vi "SSS_simulator.vi"() -> ()   [LabVIEW 2017]
panel:
  out "불리언":bool
  out "크기":i32
  out "배열":i32[](array[numeric])
  out "CMD_PWD_DATA":i32
  out "CMD_TVG_DATA":i32
  out "CMD_GAIN_DATA":i32
  out "CMD_RANGE_DATA":i32
  out "CMD_STOP_DATA":i32
  out "CMD_START_DATA":i32
  out "CMD_PWD":i32
  out "CMD_TVG":i32
  out "CMD_GAIN":i32
  out "CMD_RANGE":i32
  out "CMD_STOP":i32
  out "CMD_START":i32
  in  "port":u16=2500
  in  "address":string="30.0.1.18"
  in  "Server Closed":string="The server VI closed the connection."
  in  "TCP_Stop":bool
  # "TCP_Stop"
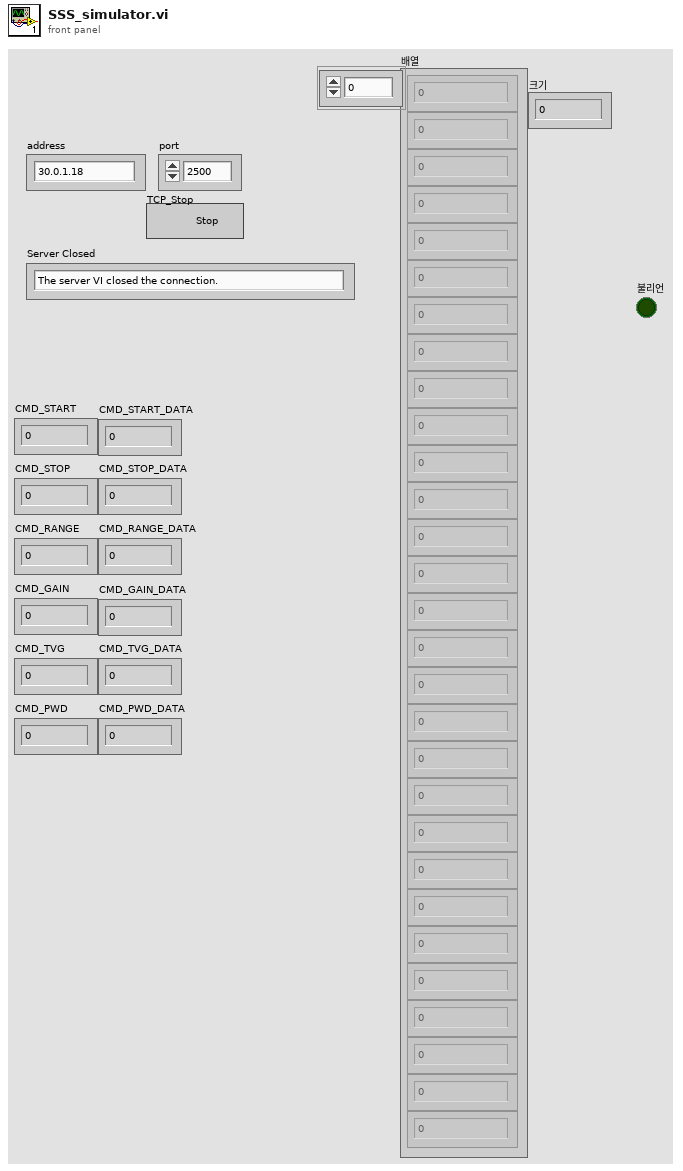
[diagram p1: front panel]
types:
  T1 = enum16{"Standard", "Buffered", "CRLF", "Immediate"}
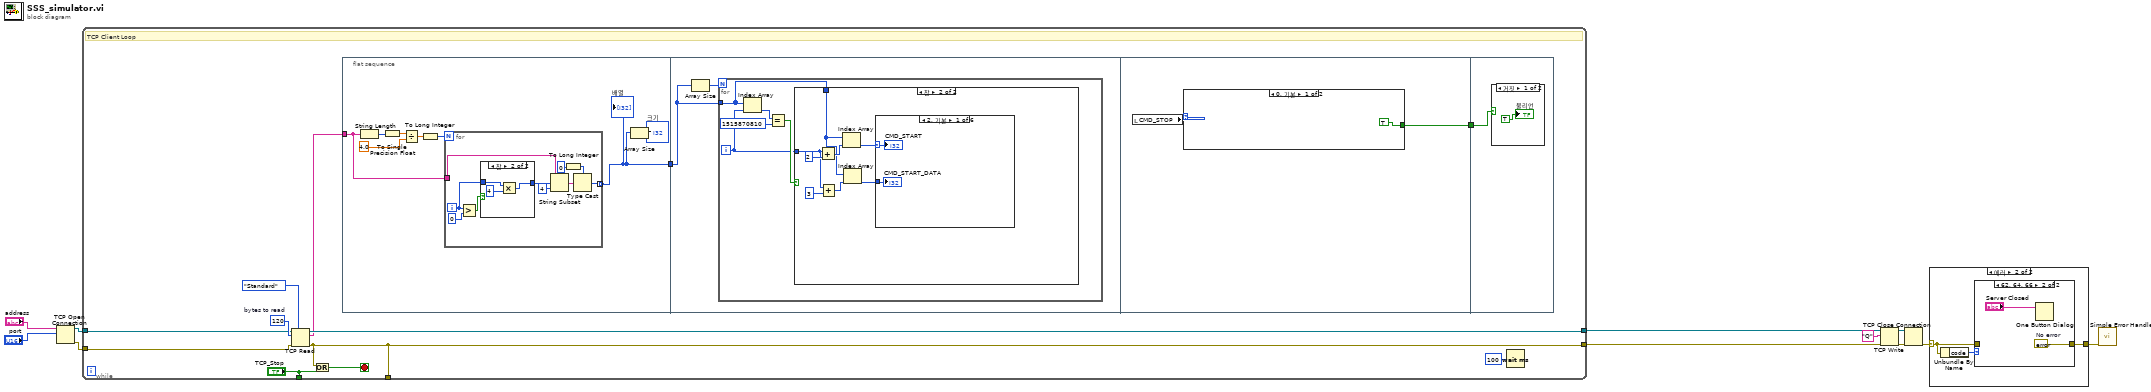
[diagram p0: block diagram]
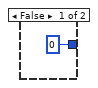
[diagram p2: hidden frame]
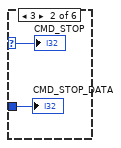
[diagram p4: hidden frame]
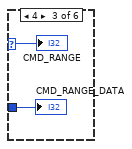
[diagram p5: hidden frame]
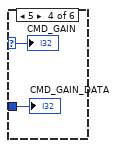
[diagram p6: hidden frame]
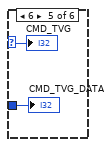
[diagram p7: hidden frame]
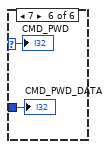
[diagram p8: hidden frame]
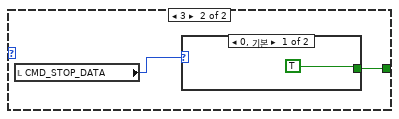
[diagram p9: hidden frame]
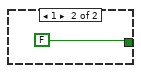
[diagram p10: hidden frame]
diagram:
  n1 = TCP Open Connection(address="address", remote port or service name="port") -> (connection ID=w1:refnum<k5>, error out=w2:errorcluster)  [unwired: 3 in]
  n2 = while {
    tunnel: [w21] -> w10
    tunnel: [w18] -> w8
    tunnel: ["TCP_Stop"] -> _
    tunnel: [w18] -> _
    tunnel: w2 -> [w15]
    tunnel: w1 -> [w14]
    stop <- w22 stop-if-true
    w23 = 120  # bytes to read
    # "TCP Client Loop"
    n3 = TCP Read(connection ID=w14, bytes to read=w23, error in (no error)=w15, 7:T1."Standard" ("모드(standard)")) -> (connection ID out=w21:refnum<k5>, data out=w16:string, error out=w18:errorcluster)  [unwired: 1 in]
    n4 = Or(x=w18, y="TCP_Stop") -> (x .or. y?=w22:bool)
    n5 = flat-sequence {
      tunnel: w16 -> [w27]
      tunnel: [w25] -> w20
      tunnel: w20 -> [w46]
      tunnel: [w73] -> w13
      tunnel: w13 -> [w80]
      frame #0 {
        n6 = String Length(string=w27) -> (length=w31:i32)
        n7 = To Single Precision Float(number=w31) -> (single precision float=w30:sgl)
        n8 = Divide(x=w30, y=sgl 4.0) -> (x/y=w28:sgl)
        n9 = To Long Integer(number=w28) -> (32bit integer=w26:i32)
        n10 = for {
          N: w26 -> [_]
          tunnel: w27 -> [w41]
          tunnel: [w38] -> w25 mode=indexing
          i -> [w33]
          n11 = Greater?(x=w33, y=0) -> (0:w35:bool)
          n12 = case shown="참" w35 {
            tunnel: [0 w43] -> w34
            tunnel: w33 -> [_ w45]
            frame False {
            }
            frame True {
              n13 = Multiply(x=w45, y=4) -> (x*y=w43:i32)
            }
          }
          n14 = String Subset(string=w41, offset (0)=w34, length (rest)=4 ("길이(나머지)")) -> (substring=w32:string)
          n15 = To Long Integer(number=0 ("숫자")) -> (32bit integer=w40:i32)
          n16 = Type Cast(type=w40, x=w32) -> (*(type *) &x=w38:i32)
        }
        "배열" <- w25
        n17 = Array Size(array=w25) -> (size(s)=→"크기":i32)
      }
      frame #1 {
        n18 = Array Size(array=w46) -> (size(s)=w47:i32)
        n19 = for {
          N: w47 -> [_]
          tunnel: w46 -> [w49]
          i -> [w48]
          n20 = Index Array(array=w49, index=w48) -> (element=w52:i32)
          n21 = Equal?(x=w52, y=1515870810) -> (x = y?=w50:bool)
          n22 = case shown="참" w50 {
            tunnel: w49 -> [_ w54]
            tunnel: w48 -> [_ w55]
            frame False {
            }
            frame True {
              n23 = Add(x=w55, y=2) -> (x+y=w59:i32)
              n24 = Add(x=w55, y=3) -> (x+y=w56:i32)
              n25 = Index Array(array=w54, index=w59) -> (element=w58:i32)
              n26 = Index Array(array=w54, index=w56) -> (element=w53:i32)
              n27 = case shown="2, 기본" w58 {
                selector: w58 -> [w62 w64 w66 w68 w70 w72]
                tunnel: w53 -> [w61 w63 w65 w67 w69 w71]
                frame 2, Default {
                  "CMD_START" <- w62
                  "CMD_START_DATA" <- w61
                }
                frame 3 {
                  "CMD_STOP" <- w64
                  "CMD_STOP_DATA" <- w63
                }
                frame 4 {
                  "CMD_RANGE" <- w66
                  "CMD_RANGE_DATA" <- w65
                }
                frame 5 {
                  "CMD_GAIN" <- w68
                  "CMD_GAIN_DATA" <- w67
                }
                frame 6 {
                  "CMD_TVG" <- w70
                  "CMD_TVG_DATA" <- w69
                }
                frame 7 {
                  "CMD_PWD" <- w72
                  "CMD_PWD_DATA" <- w71
                }
              }
            }
          }
        }
      }
      frame #2 {
        n28 = local read "CMD_STOP"() -> (w74:i32)
        n29 = case shown="0, 기본" w74 {
          tunnel: [TRUE w76] -> w73
          frame 0, Default {
          }
          frame 3 {
            n30 = local read "CMD_STOP_DATA"() -> (w77:i32)
            n31 = case shown="0, 기본" w77 {
              tunnel: [TRUE FALSE] -> w76
              frame 0, Default {
              }
              frame 1 {
              }
            }
          }
        }
      }
      frame #3 {
        n32 = case shown="거짓" w80 {
          frame False {
            "불리언" <- TRUE
          }
          frame True {
          }
        }
      }
    }
    n33 = Wait (ms)(milliseconds to wait=u32 100 ("대기 시간 (ms)")) -> ()  [unwired: 1 out]
  }
  n34 = TCP Write(connection ID=w10, data in="Q", error in (no error)=w8) -> (connection ID out=w11:refnum<k5>, error out=w9:errorcluster)  [unwired: 2 out]
  n35 = TCP Close Connection(connection ID=w11, error in (no error)=w9) -> (error out=w6:errorcluster)  [unwired: 1 in, 1 out]
  n36 = case shown="에러" w6 {
    selector: w6 -> [w82 w84]
    tunnel: [w82 w83] -> w5
    frame No Error {
    }
    frame Error {
      n37 = Unbundle By Name(w84) -> ("code"=w85:i32)
      n38 = case shown="62, 64, 66" w85 {
        tunnel: w84 -> [w86 _]
        tunnel: [w86 w88] -> w83
        frame Default {
        }
        frame 62, 64, 66 {
          w88 = errorcluster {"status"=FALSE, "code"=0, "source"=""}  # No error
          n39 = One Button Dialog(message="Server Closed") -> ()  [unwired: 1 in, 1 out]
        }
      }
    }
  }
  n40 = call <vilib>:"Simple Error Handler.vi"("error in (no error)"=w5) -> ()  [unwired: 4 in, 5 out]
